vi "Write Limit_Regex.vi"(8 "error in (no error)":errorcluster, 10 "Limit/Regex":string, 11 "String Compare in":refnum<class "String Compare.lvclass">) -> (0 "error out":errorcluster, 3 "String Compare out":refnum<class "String Compare.lvclass">)   [LabVIEW 2015, in "String Compare.lvclass"]
uses:
  String Compare.lvclass
  String Compare.lvclass/String Compare.ctl
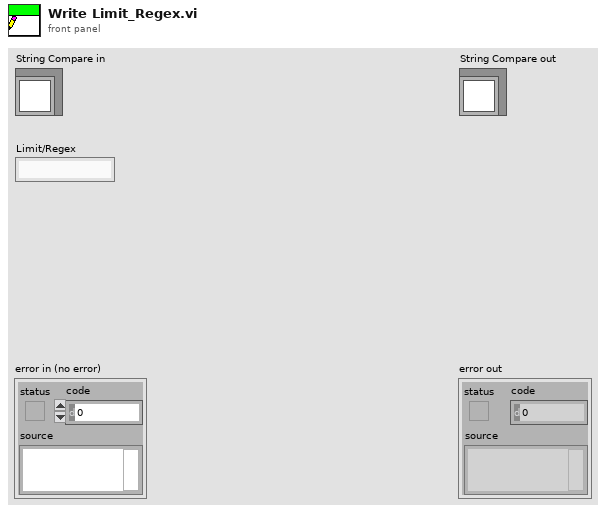
[diagram p1: front panel]
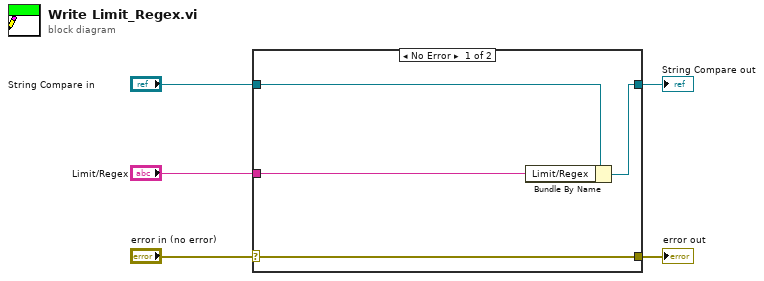
[diagram p0: block diagram]
diagram:
  n1 = case shown="No Error" "error in (no error)" {
    selector: "error in (no error)" -> [w9 w10]
    tunnel: [w9 w10] -> w4
    tunnel: [w7 w11] -> w2
    tunnel: "String Compare in" -> [w8 w11]
    tunnel: "Limit/Regex" -> [w6 _]
    frame No Error {
      n2 = Bundle By Name(cluster=w8, "Limit/Regex"=w6) -> (w7:refnum<class "String Compare.lvclass">)
    }
    frame Error {
    }
  }
  "error out" <- w4
  "String Compare out" <- w2
